vi "Close_Test.vi"(8 "error in (no error)":errorcluster caption="entrée d'erreur (pas d'erreur)", 11 "Test (Default) en entrée":refnum<class "Sequencer_With_Firebase.lvclass">) -> (0 "error out":errorcluster caption="sortie d'erreur", 3 "Test (Default) en sortie":refnum<class "Sequencer_With_Firebase.lvclass">)   [LabVIEW 2020, in "Library Core.lvlib" / "Sequencer_With_Firebase.lvclass"]
uses:
  Sequencer_With_Firebase.lvclass
  C:/Users/ngarcin/OneDrive - Altyor/Standard TB/Suite TB45/Class/Sequencer/Sequencer (Default)/Sequencer (Default).lvclass
  Commun VI/TypeDef/Variable Printable.ctl
  Creation_SN/Creation_SN Database (Default)/Creation_SN Database (Default).lvclass
  Sequencer (Default)/Sequencer (Default).lvclass
  Commun VI/Library Commun.lvlib
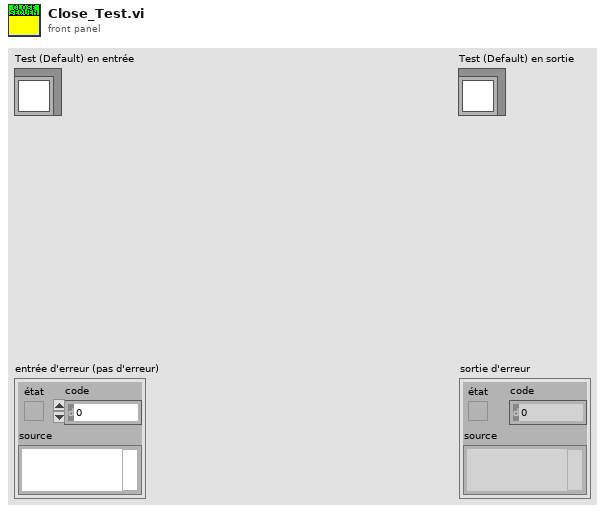
[diagram p1: front panel]
types:
  T1 = typedef "Variable Printable.ctl" = string
  T2 = enum16{"Get Variable", "Get All Variables", "Set Variable", "Delete Variable", "Delete All Variable"}
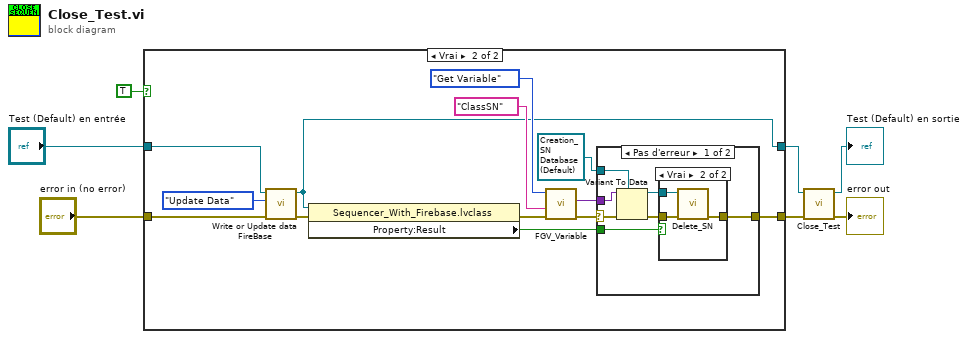
[diagram p0: block diagram]
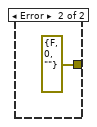
[diagram p4: hidden frame]
diagram:
  n1 = case shown="Vrai" TRUE {
    tunnel: "Test (Default) en entrée" -> [w9 w13]
    tunnel: [w8 w12] -> w4
    tunnel: [w9 w11] -> w3
    tunnel: "error in (no error)" -> [w8 w10]
    frame False {
    }
    frame True {
      n2 = call-dynamic "Write or Update data FireBase.vi"("error in (no error)"=w10, "Function"=enum16{"Set Data", "Update Data"}."Update Data", "Sequencer IN"=w13) -> ("error out"=w17:errorcluster, "Sequencer Out"=w11:refnum<class "Sequencer_With_Firebase.lvclass">)  [unwired: 7 in]
      n3 = property class="Sequencer_With_Firebase.lvclass"(reference=w11, error in=w17) -> (error out=w15:errorcluster, "Property:Result"=w16:bool)  [unwired: 1 out]
      n4 = call "FGV_Variable.vi"("error in (no error)"=w15, "Variable"=T1 "ClassSN", "Function"=T2."Get Variable") -> ("error out"=w14:errorcluster, "Data Out"=w19:variant)  [unwired: 6 in, 1 out]
      n5 = case shown="Pas d'erreur" w14 {
        selector: w14 -> [w23 _]
        tunnel: w19 -> [w29 _]
        tunnel: refnum<class "Creation_SN Database (Default).lvclass"> refnum ("Library Creation_SN.lvlib:Creation_SN Database (Default).lvclass") -> [w28 _]
        tunnel: [w25 errorcluster {"status"=FALSE, "code"=0, "source"=""} ("error out")] -> w12
        tunnel: w16 -> [w24 _]
        frame No Error {
          n6 = Variant To Data(error in=w23, type=w28, Variant=w29) -> (data=w26:refnum<class "Creation_SN Database (Default).lvclass">, error out=w27:errorcluster)
          n7 = case shown="Vrai" w24 {
            tunnel: w27 -> [w30 w33]
            tunnel: w26 -> [_ w32]
            tunnel: [w30 w31] -> w25
            frame False {
            }
            frame True {
              n8 = call-dynamic "Delete_SN.vi"("error in (no error)"=w33, "Class Creation_SN (Default) en entrée"=w32) -> ("error out"=w31:errorcluster)  [unwired: 8 in, 1 out]
            }
          }
        }
        frame Error {
        }
      }
    }
  }
  n9 = call-parent "Close_Test.vi"("error in (no error)"=w4, "Test (Default) en entrée"=w3) -> ("error out"=→"error out":errorcluster, "Test (Default) en sortie"=→"Test (Default) en sortie":refnum<class "Sequencer_With_Firebase.lvclass">)  [unwired: 8 in]
